vi "ScanrangeY.vi"() -> ()   [LabVIEW 2013]
panel:
  in  "Scanrange Y":dbl format="%.2f"
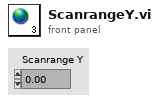
[diagram p1: front panel]
diagram:
